vi "DIO_port.vi"() -> ()   [LabVIEW 2021]
uses:
  <vilib>/rvi/eio/common/nirviEmuTemplateMethod_errors.vi
  <vilib>/eio/EIONode/EIONode.xnode
panel:
  out "number":u8
  in  "DO 7:0":bool[](array[boolean])=[FALSE, FALSE, FALSE, FALSE, FALSE, FALSE, FALSE, FALSE]
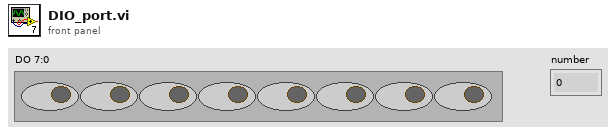
[diagram p1: front panel]
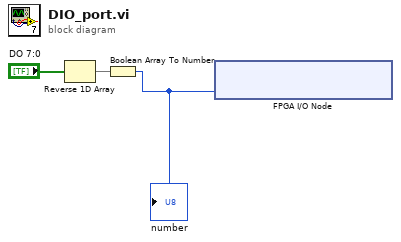
[diagram p0: block diagram]
diagram:
  n1 = Reverse 1D Array(array="DO 7:0") -> (reversed array=w3:bool[])
  n2 = Boolean Array To Number(Boolean array=w3) -> (number=w1:u8)
  "number" <- w1
  n3 = xnode "FPGA I/O Node"("Connector0/DIOPORT0"=w1) -> ()  [unwired: 1 in, 1 out]
